vi "数据查询_仪器数据.vi"() -> ()   [LabVIEW 2016]
uses:
  <vilib>/Utility/miscctls.llb/LVPositionTypeDef.ctl
  <vilib>/Utility/miscctls.llb/LVRowAndColumnUnsignedTypeDef.ctl
  <vilib>/Utility/miscctls.llb/LVPointTypeDef.ctl
  <userlib>/_OpenG.lib/array/array.llb/Sort 2D Array (String)__ogtk.vi
  <userlib>/_OpenG.lib/array/array.llb/Sort 1D Array (I32)__ogtk.vi
  <vilib>/regexp/Match Regular Expression.xnode
panel:
  in  "触发查询":bool
  out "位置 2":T1 caption="位置"
  out "位置":T1
  out "condition":string
  out "显示项":string[](array[string])
  out "确定查询":bool
  in  "布尔":bool
  in  "条件筛选":bool
  in  "数据列表选择框":string(xcontrol)
  in  "导出":bool
  in  "数据表":T2
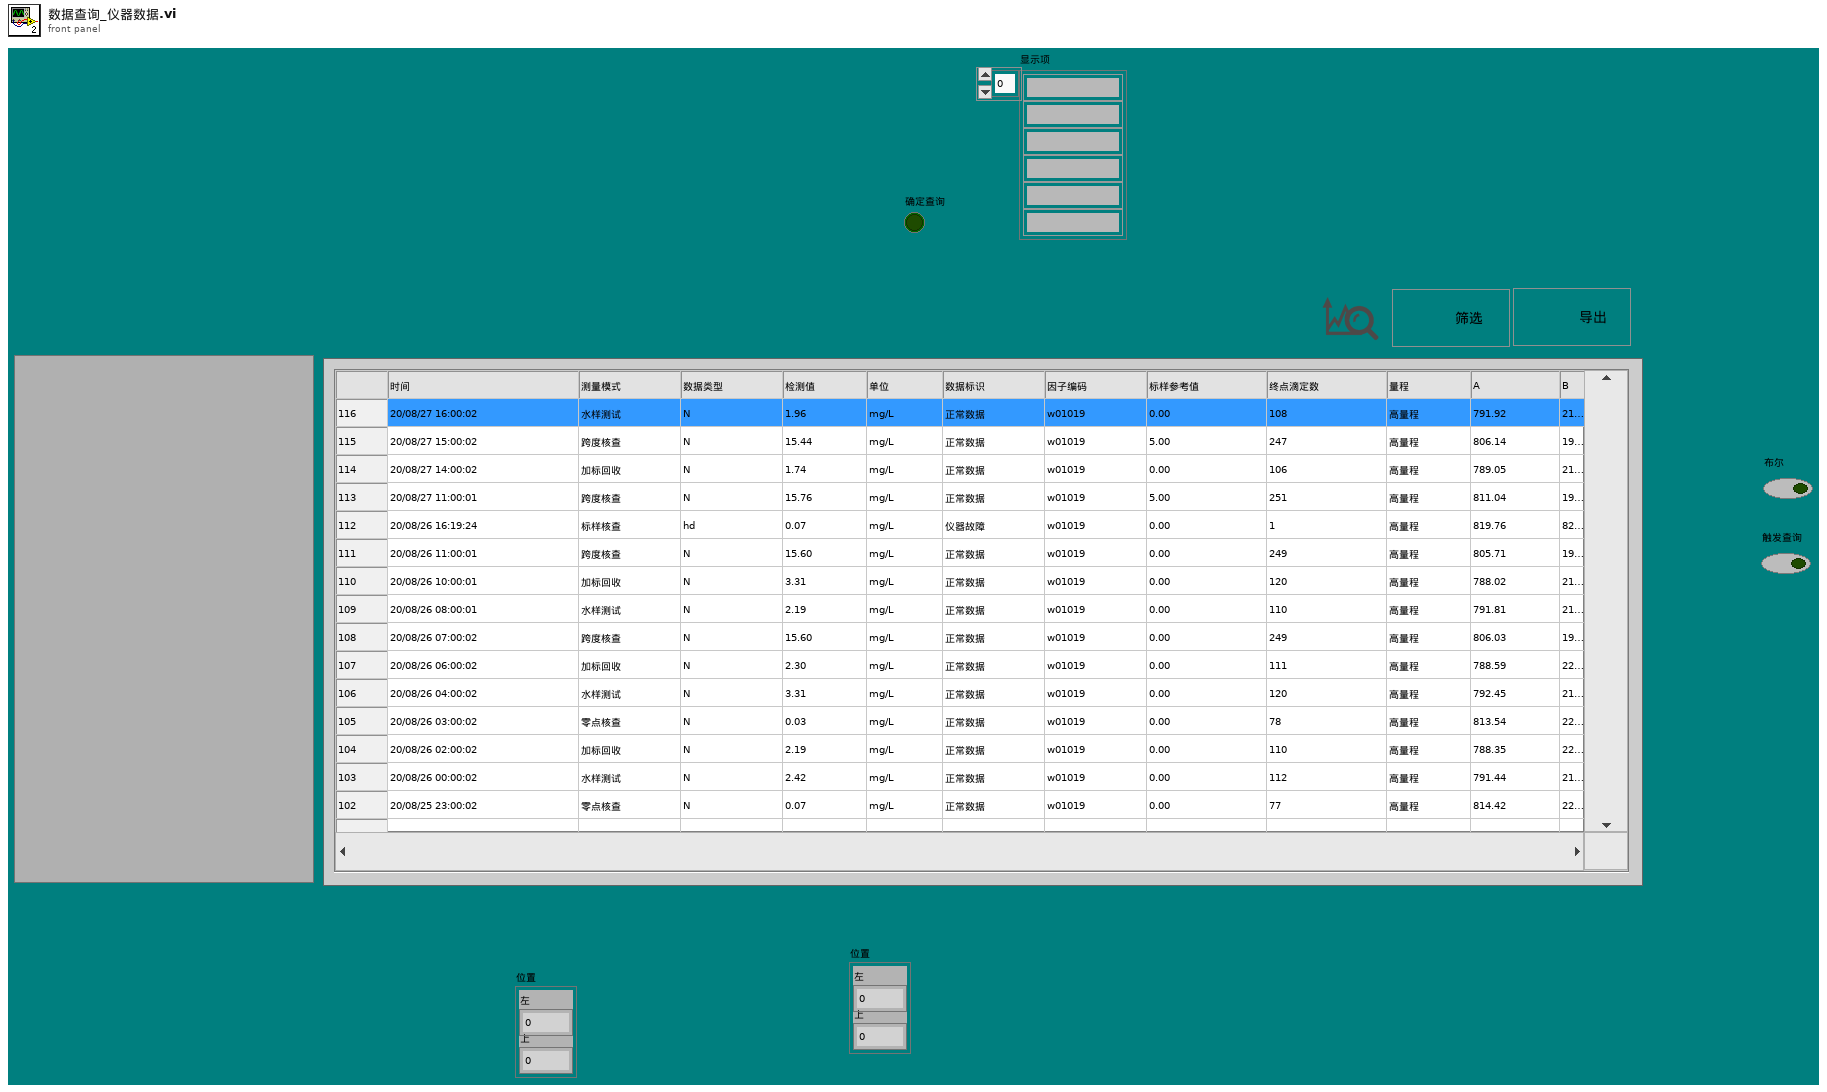
[diagram p1: front panel]
types:
  T1 = typedef "LVPositionTypeDef.ctl" = cluster{"Left":i32, "Top":i32}
  T2 = typedef "数据查询大列表框.ctl" = i32
  T3 = typedef "LVRowAndColumnUnsignedTypeDef.ctl" = cluster{"Row":u32, "Column":u32}
  T4 = typedef "LVPointTypeDef.ctl" = cluster{"Horizontal":i16, "Vertical":i16}
  T5 = enum8{"Enabled", "Disabled", "Disabled and Grayed Out"}
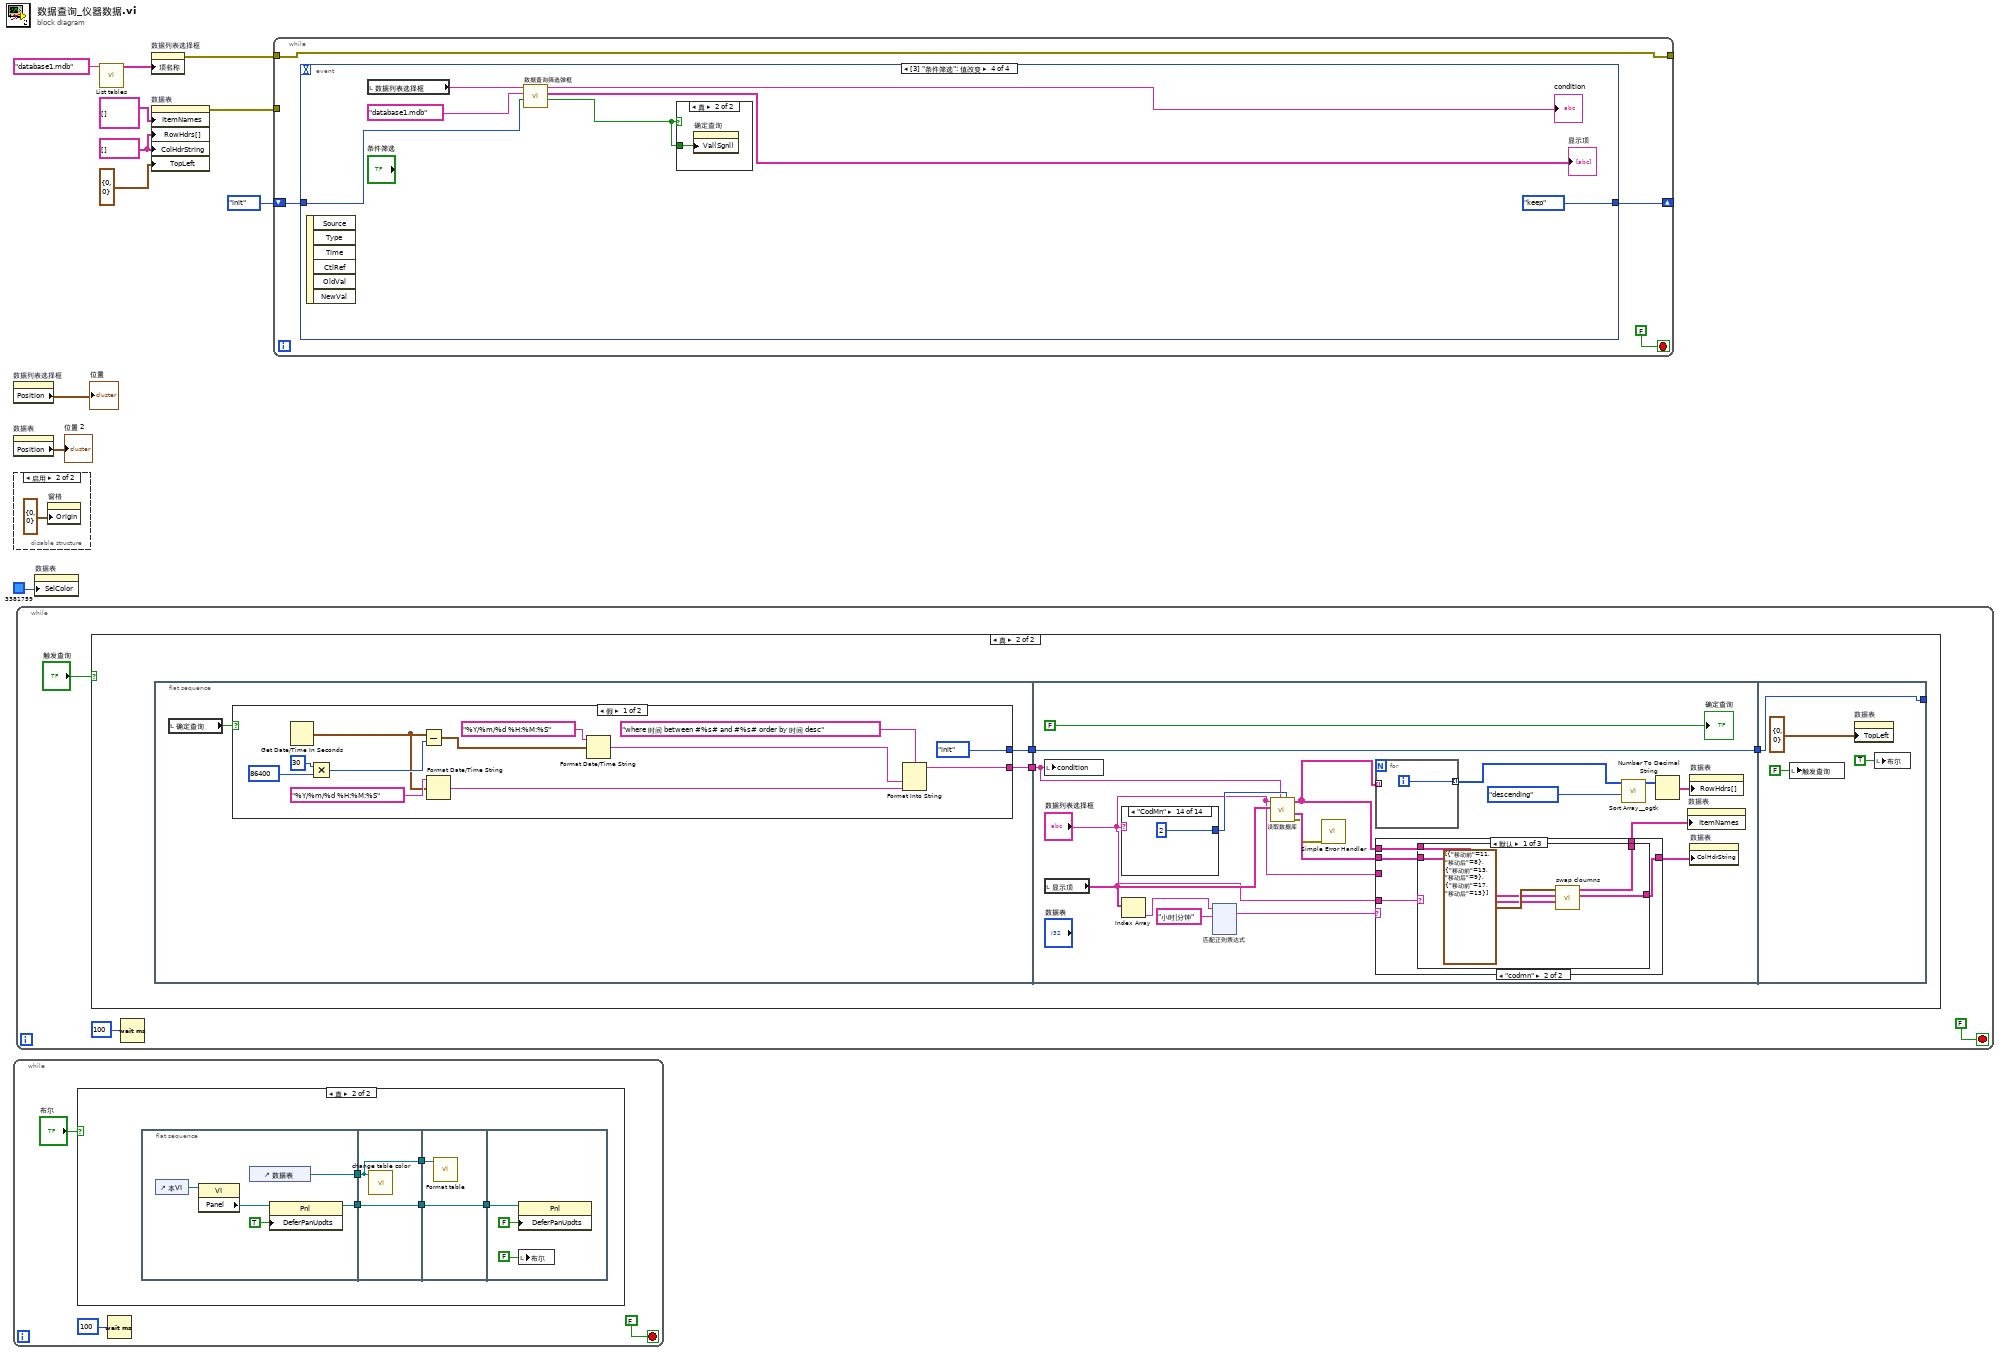
[diagram p0: block diagram]
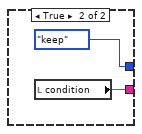
[diagram p3: hidden frame]
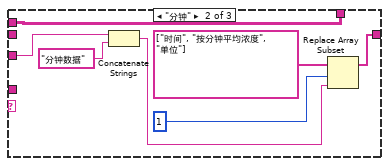
[diagram p5: hidden frame]
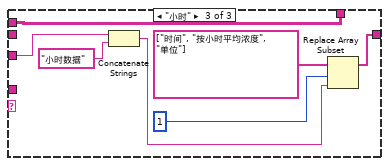
[diagram p6: hidden frame]
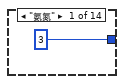
[diagram p7: hidden frame]
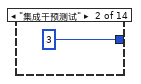
[diagram p8: hidden frame]
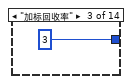
[diagram p9: hidden frame]
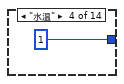
[diagram p10: hidden frame]
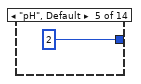
[diagram p11: hidden frame]
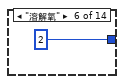
[diagram p12: hidden frame]
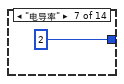
[diagram p13: hidden frame]
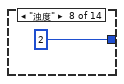
[diagram p14: hidden frame]
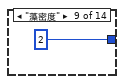
[diagram p15: hidden frame]
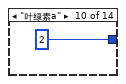
[diagram p16: hidden frame]
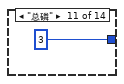
[diagram p17: hidden frame]
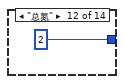
[diagram p18: hidden frame]
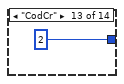
[diagram p19: hidden frame]
diagram:
  w8 = string[] [] ("行首字符串[]")
  n1 = property on="数据列表选择框" class="数据列表选择框 (严格)"() -> ("Position"=→"位置":T1)  [unwired: 2 in, 2 out]
  n2 = property on="数据表" class="MCListbox (严格)"() -> ("Position"=→"位置 2":T1)  [unwired: 2 in, 2 out]
  n3 = disable-structure shown="启用" {
    frame Disabled {
    }
    frame Enabled {
      n4 = property on="窗格" class="Pane"("Origin"=T4 {"Horizontal"=0, "Vertical"=0} ("原点")) -> ()  [unwired: 2 in, 2 out]
    }
  }
  n5 = while {
    stop <- FALSE stop-if-true
    n6 = case shown="真" "布尔" {
      frame False {
      }
      frame True {
        n7 = flat-sequence {
          tunnel: [w22] -> w18
          tunnel: [w21] -> w17
          tunnel: [w27] -> w19
          tunnel: w18 -> [w27]
          tunnel: w17 -> [w26]
          tunnel: [w26] -> w16
          tunnel: [w29] -> w20
          tunnel: w19 -> [w29]
          tunnel: w16 -> [w28]
          tunnel: w20 -> [w32]
          frame #0 {
            n8 = control-ref of="本VI"() -> (w23:refnum<vi>)
            n9 = property class="VI"(reference=w23) -> ("Panel"=w24:refnum<vi>)  [unwired: 1 in, 2 out]
            n10 = control-ref of="数据表"() -> (w21:refnum<vi>)
            n11 = property class="Pnl"(reference=w24, "DeferPanUpdts"=TRUE ("延迟前面板更新")) -> (reference out=w22:refnum<vi>)  [unwired: 1 in, 1 out]
          }
          frame #1 {
            n12 = call "change table color.vi"("MulticolumnListbox输入"=w26) -> ()  [unwired: 11 in]
          }
          frame #2 {
            n13 = call "Format table.vi"("Table输入"=w28) -> ()  [unwired: 11 in]
          }
          frame #3 {
            n14 = property class="Pnl"(reference=w32, "DeferPanUpdts"=FALSE ("延迟前面板更新")) -> ()  [unwired: 1 in, 2 out]
            n15 = local write "布尔"(FALSE ("布尔")) -> ()
          }
        }
      }
    }
    n16 = Wait (ms)(milliseconds to wait=u32 100 ("等待时间（毫秒）")) -> ()  [unwired: 1 out]
  }
  n17 = while {
    stop <- FALSE stop-if-true
    n18 = case shown="真" "触发查询" {
      frame False {
      }
      frame True {
        n19 = flat-sequence {
          tunnel: [w40] -> w38
          tunnel: [w39] -> w37
          tunnel: w38 -> [w61]
          tunnel: [w60] -> w36
          tunnel: w37 -> [w60]
          tunnel: [w230] -> _
          tunnel: w36 -> [w230]
          frame #0 {
            n20 = local read "确定查询"() -> (w41:bool)
            n21 = case shown="假" w41 {
              tunnel: [w44 w55] -> w40
              tunnel: [enum16{"init", "keep"}."init" ("是否初始化") enum16{"init", "keep"}."keep" ("是否初始化")] -> w39
              frame False {
                n22 = Get Date/Time In Seconds() -> (seconds since 1Jan1904=w42:timestamp)
                n23 = Multiply(x=30, y=86400) -> (x*y=w45:i32)
                n24 = Subtract(x=w42, y=w45) -> (x-y=w50:timestamp)
                n25 = Format Date/Time String(time format string (%c)="%Y/%m/%d %H:%M:%S" ("时间格式字符串(%c)"), seconds (now)=w42) -> (date/time string=w53:string)  [unwired: 1 in]
                n26 = Format Date/Time String(time format string (%c)="%Y/%m/%d %H:%M:%S" ("时间格式字符串(%c)"), seconds (now)=w50) -> (date/time string=w52:string)  [unwired: 1 in]
                n27 = Format Into String(format string="where 时间 between #%s# and #%s# order by 时间 desc", w52, w53) -> (resulting string=w44:string)  [unwired: 2 in, 1 out]
              }
              frame True {
                n28 = local read "condition"() -> (w55:string)
              }
            }
          }
          frame #1 {
            n29 = local write "condition"(w61) -> ()
            n30 = local read "显示项"() -> (w66:string[])
            n31 = case shown="\"CodMn\"" "数据列表选择框" {
              tunnel: [i16 3 ("精度(6)") i16 3 ("精度(6)") i16 3 ("精度(6)") i16 1 ("精度(6)") i16 2 ("精度(6)") i16 2 ("精度(6)") i16 2 ("精度(6)") i16 2 ("精度(6)") i16 2 ("精度(6)") i16 2 ("精度(6)") i16 3 ("精度(6)") i16 2 ("精度(6)") i16 2 ("精度(6)") i16 2 ("精度(6)")] -> w71
              frame "氨氮" {
              }
              frame "集成干预测试" {
              }
              frame "加标回收率" {
              }
              frame "水温" {
              }
              frame "pH", Default {
              }
              frame "溶解氧" {
              }
              frame "电导率" {
              }
              frame "浊度" {
              }
              frame "藻密度" {
              }
              frame "叶绿素a" {
              }
              frame "总磷" {
              }
              frame "总氮" {
              }
              frame "CodCr" {
              }
              frame "CodMn" {
              }
            }
            n32 = Index Array(array=w66) -> (element=w64:string)  [unwired: 1 in]
            n33 = xnode "匹配正则表达式"("输入字符串"=w64, "正则表达式"="小时|分钟") -> ("所有匹配"=w63:string)  [unwired: 4 in, 4 out]
            n34 = call "读取数据库.vi"("精度(6)"=w71, "condition"=w61, "显示项"=w66, "组合框"="数据列表选择框") -> ("error out"=w59:errorcluster, "columns"=w70:string[], "表格"=w58:string[][])  [unwired: 4 in, 1 out]
            n35 = call <vilib>:"Simple Error Handler.vi"("error in (no error)"=w59) -> ()  [unwired: 4 in, 5 out]
            n36 = for {
              tunnel: w58 -> [_] mode=indexing
              tunnel: [w228] -> w73 mode=indexing
              i -> [w228]
            }
            n37 = case shown="默认" w63 {
              tunnel: w70 -> [w190 _ _]
              tunnel: [w188 w204 w209] -> w69
              tunnel: "数据列表选择框" -> [_ w203 w210]
              tunnel: w58 -> [w191 w200 w207]
              tunnel: [w189 w200 w207] -> w57
              tunnel: "数据列表选择框" -> [w192 _ _]
              frame Default {
                n38 = case shown="\"codmn\"" w192 {
                  tunnel: w191 -> [w194 w198]
                  tunnel: w190 -> [w193 w197]
                  tunnel: [w194 w196] -> w189
                  tunnel: [w193 w195] -> w188
                  frame "假", Default {
                  }
                  frame "codmn" {
                    n39 = call "swap cloumns.vi"("columns"=w197, "表格"=w198, "交换参数"=cluster{"移动前":i32, "移动后":i32}[] [{"移动前"=11, "移动后"=8}, {"移动前"=13, "移动后"=9}, {"移动前"=17, "移动后"=13}]) -> ("columns 2"=w195:string[], "表格 2"=w196:string[][])  [unwired: 7 in]
                  }
                }
              }
              frame "分钟" {
                n40 = Concatenate Strings(w203, "分钟数据" ("字符串")) -> (w201:string)
                n41 = Replace Array Subset(array=string[] ["时间", "按分钟平均浓度", "单位"] ("columns"), new element=w201, index=1 ("索引")) -> (w204:string[])
              }
              frame "小时" {
                n42 = Concatenate Strings(w210, "小时数据" ("字符串")) -> (w211:string)
                n43 = Replace Array Subset(array=string[] ["时间", "按小时平均浓度", "单位"] ("columns"), new element=w211, index=1 ("索引")) -> (w209:string[])
              }
            }
            n44 = call-poly <userlib>:"Sort Array__ogtk.vi"("Order"=enum16{"ascending", "descending"}."descending", "Array in"=w73) -> ("Sorted Array out"=w67:i32[])  [unwired: 8 in, 1 out]
            n45 = Number To Decimal String(number=w67) -> (decimal integer string=w72:string[])  [unwired: 1 in]
            n46 = property on="数据表" class="MCListbox (严格)"("ItemNames"=w57) -> ()  [unwired: 2 in, 2 out]
            n47 = property on="数据表" class="MCListbox (严格)"("RowHdrs[]"=w72) -> ()  [unwired: 2 in, 2 out]
            n48 = property on="数据表" class="MCListbox (严格)"("ColHdrString"=w69) -> ()  [unwired: 2 in, 2 out]
            "确定查询" <- FALSE ("确定查询")
          }
          frame #2 {
            n49 = local write "触发查询"(FALSE ("触发查询")) -> ()
            n50 = property on="数据表" class="MCListbox (严格)"("TopLeft"=T3 {"Row"=0, "Column"=0} ("索引值")) -> ()  [unwired: 2 in, 2 out]
            n51 = local write "布尔"(TRUE ("布尔")) -> ()
          }
        }
      }
    }
    n52 = Wait (ms)(milliseconds to wait=u32 100 ("等待时间（毫秒）")) -> ()  [unwired: 1 out]
  }
  n53 = property on="数据表" class="MCListbox (严格)"("SelColor"=u32 3381759) -> ()  [unwired: 2 in, 2 out]
  n54 = call "List tables.vi"("database"="database1.mdb") -> ("tables"=w6:string[])  [unwired: 9 in, 1 out]
  n55 = property on="数据列表选择框" class="数据列表选择框 (严格)"("项名称"=w6) -> (error out=w4:errorcluster)  [unwired: 2 in, 1 out]
  n56 = property on="数据表" class="MCListbox (严格)"("ItemNames"=string[][] [] ("项名"), "RowHdrs[]"=w8, "ColHdrString"=w8, "TopLeft"=T3 {"Row"=0, "Column"=0} ("左上可见单元格")) -> (error out=w10:errorcluster)  [unwired: 2 in, 1 out]
  n57 = while {
    tunnel: w10 -> [_]
    tunnel: [w235] -> _
    tunnel: w4 -> [w235]
    shift-right: [w233] -> _
    shift-left: enum16{"init", "keep"}."init" ("是否初始化") -> [w234]
    stop <- FALSE stop-if-true
    n58 = event shown="[3] \"条件筛选\": 值改变" {
      selector: _ -> [_ _ _ _]
      dyn-events: _ -> [_ _ _ _]
      timeout: _ -> [_ _ _ _]
      tunnel: w234 -> [_ _ _ w279]
      tunnel: [_ enum16{"init", "keep"}."keep" ("是否初始化") w272 enum16{"init", "keep"}."keep" ("是否初始化")] -> w233
      event Timeout {
        n59 = event-data() -> ()  [unwired: 1 in, 3 out]
      }
      event "导出": Value Change {
        n60 = event-data() -> ("CtlRef"=w238:refnum<vi>)  [unwired: 1 in, 5 out]
        n61 = property class="Bool"(reference=w238, "DisabledEnum"=T5."Disabled and Grayed Out" ("禁用")) -> (reference out=w242:refnum<vi>, error out=w243:errorcluster)  [unwired: 1 in]
        n62 = flat-sequence {
          tunnel: w243 -> [_]
          tunnel: [w260] -> w241
          tunnel: w242 -> [w260]
          tunnel: "导出" -> [_]
          frame #0 {
            n63 = property on="数据表" class="MCListbox (严格)"() -> ("ColHdrString"=w247:string[])  [unwired: 2 in, 2 out]
            n64 = Array Size(array=w247) -> (size(s)=w254:i32)
            n65 = property on="数据表" class="MCListbox (严格)"() -> ("ItemNames"=w245:string[][])  [unwired: 2 in, 2 out]
            n66 = Greater Or Equal?(x=w254, y=5) -> (x >= y?=w252:bool)
            n67 = call "Removable devices detection v8.5.vi"() -> ("Removable"=w257:string[])  [unwired: 4 out]
            n68 = Select(t=3 ("禁用的索引 (列)"), s=w252, f=1) -> (s? t:f=w250:i32)
            n69 = call-poly <userlib>:"Sort Array__ogtk.vi"("Column/Row to Sort By"=u32 0, "Sort By in"=enum16{"row", "column"}."column", "Order"=enum16{"ascending", "descending"}."ascending", "Array in"=w245) -> ("Sorted Array out"=w267:string[][])  [unwired: 4 in, 3 out]
            n70 = Index Array(array=w267, index (col)=w250) -> (element=w263:string[])  [unwired: 1 in]
            n71 = Index Array(array=w257) -> (element=w256:string)  [unwired: 1 in]
            n72 = String To Path(string=w256) -> (path=w255:path)
            n73 = Get Date/Time In Seconds() -> (seconds since 1Jan1904=w268:timestamp)
            n74 = local read "数据列表选择框"() -> (w261:string)
            n75 = Fract/Exp String To Number(string=w263) -> (number=w262:dbl[])  [unwired: 3 in, 1 out]
            n76 = Insert Into Array(array=string[][] [], new element=w247) -> (w246:string[][])  [unwired: 2 in]
            n77 = call "MS Office Report"("Path to Save Report"=w255, "导出日期"=w268, "监测参数"=w261, "数据输入"=w267, "图表输入"=w262, "字段定义"=w246) -> ("error out"=w259:errorcluster)  [unwired: 20 in, 1 out]
            n78 = case shown="错误" w259 {
              tunnel: ["导出成功" ("消息") "导出失败" ("消息")] -> w258
              frame No Error {
              }
              frame Error {
              }
            }
            n79 = One Button Dialog(message=w258) -> ()  [unwired: 1 in, 1 out]
          }
        }
        n80 = property class="Bool"(reference=w241, "DisabledEnum"=T5."Enabled" ("禁用")) -> ()  [unwired: 1 in, 2 out]
      }
      event "数据列表选择框": Mouse Up; "确定查询": Value Change {
        n81 = event-data() -> ()  [unwired: 1 in, 4 out]
        n82 = call "List tables.vi"("database"="database1.mdb") -> ("tables"=w274:string[])  [unwired: 9 in, 1 out]
        n83 = property on="数据列表选择框" class="数据列表选择框 (严格)"("项名称"=w274) -> ()  [unwired: 2 in, 2 out]
        n84 = local read "确定查询"() -> (w273:bool)
        n85 = case shown="假" w273 {
          tunnel: [enum16{"init", "keep"}."init" ("是否初始化") enum16{"init", "keep"}."keep" ("是否初始化")] -> w272
          frame False {
          }
          frame True {
          }
        }
        n86 = local write "触发查询"(TRUE ("触发查询")) -> ()
      }
      event "条件筛选": Value Change {
        n87 = event-data() -> ()  [unwired: 1 in, 6 out]
        n88 = local read "数据列表选择框"() -> (w283:string)
        n89 = call "数据查询筛选弹框.vi"("是否初始化"=w279, "database"="database1.mdb", "table"=w283) -> ("确定输出"=w280:bool, "显示项"=→"显示项":string[], "condition"=→"condition":string)  [unwired: 5 in, 1 out]
        n90 = case shown="真" w280 {
          tunnel: w280 -> [_ w285]
          frame False {
          }
          frame True {
            n91 = property on="确定查询" class="Bool (严格)"("Val(Sgnl)"=w285) -> ()  [unwired: 2 in, 2 out]
          }
        }
      }
    }
  }
